vi "sm bool read and increment.vi"(8 "Identifier":string, 11 "Shared memory cluster input":T1) -> (2 "Bool out":bool, 3 "Shared memory cluster output":T1)   [LabVIEW 2018, in "linuxSharedMemory.lvlib"]
uses:
  linuxSharedMemory.lvlib
  controls/sm_cluster.ctl
  <vilib>/NI/NI Linux RT IPC/Shared Memory/Pointer Operations/Read Scalar Boolean.vi
  <vilib>/NI/NI Linux RT IPC/Shared Memory/Pointer Operations/In Place Read Pointer.vi
  <vilib>/NI/NI Linux RT IPC/Shared Memory/Pointer Operations/In Place Read Scalar Boolean.vi
  <vilib>/NI/NI Linux RT IPC/Shared Memory/Linux RT IPC.Shared Memory.lvlib
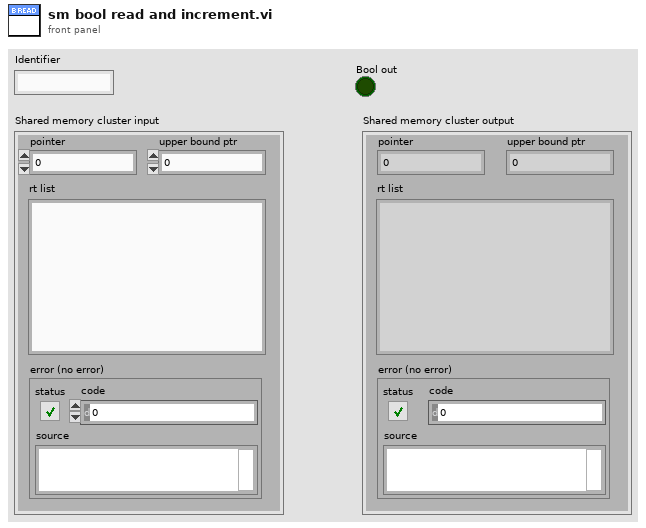
[diagram p1: front panel]
types:
  T1 = typedef "linuxSharedMemory.lvlib/sm_cluster.ctl" = cluster{"rt list":string, "error (no error)":errorcluster, "pointer":u64, "upper bound ptr":u64}
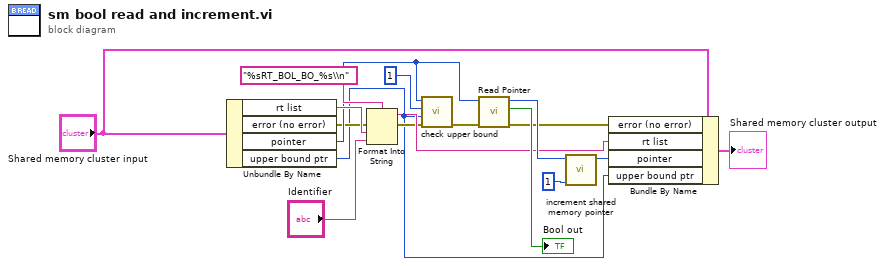
[diagram p0: block diagram]
diagram:
  n1 = Unbundle By Name("Shared memory cluster input") -> ("rt list"=w13:string, "error (no error)"=w7:errorcluster, "pointer"=w12:u64, "upper bound ptr"=w4:u64)
  n2 = Format Into String(format string="%sRT_BOL_BO_%s\\n", error in=w7, w13, "Identifier") -> (resulting string=w8:string, error out=w6:errorcluster)  [unwired: 1 in]
  n3 = call "check upper bound.vi"("error in (no error)"=w6, "ptr upper bound (inclusive)"=w4, "size"=1, "ptr in"=w12) -> ("error out"=w10:errorcluster)  [unwired: 7 in]
  n4 = call-poly <vilib>:"Read Pointer.vi"("error in (no error)"=w10, "pointer in"=w12) -> ("error out"=w9:errorcluster, "value out"=→"Bool out":bool, "pointer out"=w17:u64)  [unwired: 7 in]
  n5 = call "increment shared memory pointer.vi"("Increment value"=1, "Shared Memory PTR in"=w17) -> ("Shared Memory PTR out"=w5:u64)  [unwired: 9 in]
  n6 = Bundle By Name(cluster="Shared memory cluster input", "error (no error)"=w9, "rt list"=w8, "pointer"=w5, "upper bound ptr"=w4) -> (→"Shared memory cluster output":T1)
